vi "QI radial profile calculate_new.vi"(5 "num":i32, 7 "r":dbl, 8 "rad":dbl[](array[numeric]), 9 "Yr":dbl, 10 "Xr":dbl, 11 "ROI array":sgl[][](array[numeric])) -> (0 "mean 4":dbl, 1 "mean 3":dbl, 2 "mean 2":dbl, 3 "mean":dbl)   [LabVIEW 2017]
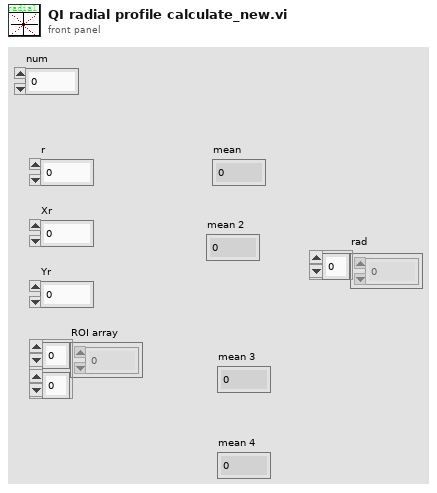
[diagram p1: front panel]
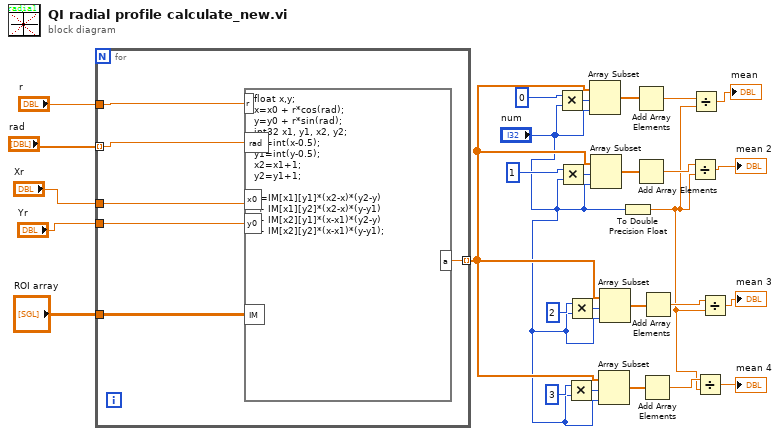
[diagram p0: block diagram]
diagram:
  n1 = for "For循环" {
    tunnel: "Xr" -> [w34]
    tunnel: "Yr" -> [w33]
    tunnel: "r" -> [w32]
    tunnel: "ROI array" -> [w29]
    tunnel: [w31] -> w15 mode=indexing
    tunnel: "rad" -> [w30] mode=indexing
    n2 = formula code="float x,y;\nx=x0 + r*cos(rad);\ny=y0 + r*sin(rad);\nint32 x1, y1, x2, y2;\nx1=int(x-0.5);\ny1=int(y-0.5);\nx2=x1+1;\ny2=y1+1;\n\na=IM[x1][y1]*(x2-x)*(y2-y)\n + IM[x1][y2]*(x2-x)*(y-y1)\n + IM[x2][y1]*(x-x1)*(y2-y)\n + IM[x2][y2]*(x-x1)*(y-y1);"("x0"=w34, "y0"=w33, "rad"=w30, "r"=w32, "IM"=w29) -> ("a"=w31:dbl)
  }
  n3 = Multiply(x=0 ("索引"), y="num") -> (x*y=w22:i32)
  n4 = Multiply(x=1 ("索引"), y="num") -> (x*y=w21:i32)
  n5 = Multiply(x=3 ("索引"), y="num") -> (x*y=w17:i32)
  n6 = Multiply(x=2 ("索引"), y="num") -> (x*y=w18:i32)
  n7 = Array Subset(array=w15, index=w22, length="num") -> (w14:dbl[])
  n8 = Array Subset(array=w15, index=w21, length="num") -> (w13:dbl[])
  n9 = Array Subset(array=w15, index=w17, length="num") -> (w11:dbl[])
  n10 = Array Subset(array=w15, index=w18, length="num") -> (w12:dbl[])
  n11 = To Double Precision Float(number="num") -> (double precision float=w3:dbl)
  n12 = Add Array Elements(numeric array=w14) -> (sum=w8:dbl)
  n13 = Add Array Elements(numeric array=w13) -> (sum=w10:dbl)
  n14 = Add Array Elements(numeric array=w11) -> (sum=w7:dbl)
  n15 = Add Array Elements(numeric array=w12) -> (sum=w6:dbl)
  n16 = Divide(x=w10, y=w3) -> (x/y=→"mean 2":dbl)
  n17 = Divide(x=w8, y=w3) -> (x/y=→"mean":dbl)
  n18 = Divide(x=w7, y=w3) -> (x/y=→"mean 4":dbl)
  n19 = Divide(x=w6, y=w3) -> (x/y=→"mean 3":dbl)
